vi "MarkWaypointComplete.vi"(2 "Error In":errorcluster, 3 "Waypoint In":refnum<class "Waypoint.lvclass">) -> (0 "Error Out":errorcluster, 1 "Waypoint Out":refnum<class "Waypoint.lvclass">)   [LabVIEW 2012, in "Waypoint.lvclass"]
uses:
  Waypoint.lvclass
  Waypoint.lvclass/Waypoint.ctl
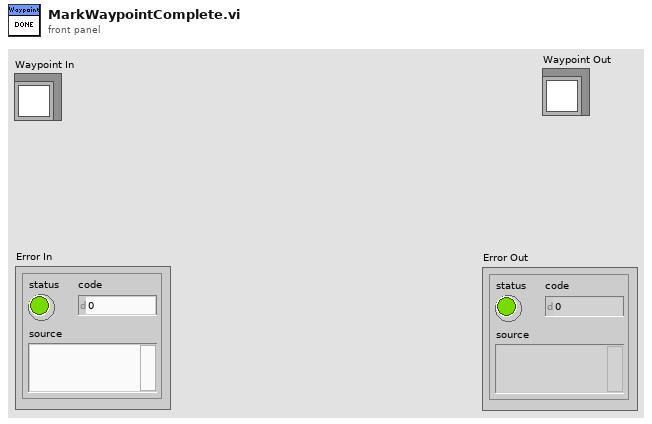
[diagram p1: front panel]
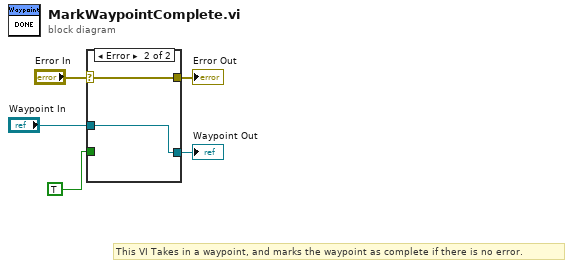
[diagram p0: block diagram]
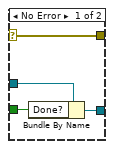
[diagram p2: hidden frame]
diagram:
  # "This VI Takes in a waypoint, and marks the waypoint as complete if there is no error."
  n1 = case shown="Error" "Error In" {
    selector: "Error In" -> [w9 w11]
    tunnel: [w9 w11] -> w4
    tunnel: "Waypoint In" -> [w8 w10]
    tunnel: [w7 w10] -> w2
    tunnel: TRUE ("Done?") -> [w6 _]
    frame No Error {
      n2 = Bundle By Name(cluster=w8, "Done?"=w6) -> (w7:refnum<class "Waypoint.lvclass">)
    }
    frame Error {
    }
  }
  "Waypoint Out" <- w2
  "Error Out" <- w4
